vi "Contrast.vi"(4 "Burst Ct":i8[](array[numeric])=[1, 3, 5, 10, 20], 6 "CA Threshold":i16=62, 8 "File Name In":string, 9 "Voltage Steps":sgl[](array[numeric])=[100.0] format="%_3g", 10 "Motion Settings":T1={"No Motion?"=FALSE, "Motion System"=enum."NI 735x", "Motion Bd ID"=1, "Motion Profile"="SMAC1", "# Axis"=1, "Reverse Z axis?"=TRUE, "SMAC Axis"=0, "scan pair"=enum."y-(x) scan", "RT fps"=6.0, "Steps per mm"=[1000, 1000, 1000, 1000], "Motor Parameters"={"velocity ct/s"=[10000.0, 10000.0, 10000.0, 50000.0], "accel ct/s^2"=[50000.0, 50000.0, 50000.0, 200000.0]}, "One Way Scan"=FALSE, "Reverse One Way Scan"=FALSE, "Global Position (mm)"=[], "Plane"=0, "Distance between\nscan lines (um)"=0.0, "Distance between\nscan planes (um)"=0.0, "number of scan planes"=1, "Total steps in line"=0, "Xtra plane\ndistance  (um)"=100, "Xtra planes "=1, "Add Axis"=FALSE, "overshoot cts"=200, "BKPT Shift"=0, "Scan Start Time (ms)"=0, "ESP VISA"="GPIB::1::INSTR", "3rd Axis"=1, "GL Ref Out"=refnum, "Galil Address"=""} {"3rd Axis" items=["x", "y", "z", "w"]; "Xtra planes" min=1; "Xtra plane\ndistance  (um)" min=0; "Distance between\nscan planes (um)" format="%.2f"; "Distance between\nscan lines (um)" format="%.2f"; "SMAC Axis" items=["None"=0, "Axis 1"=1, "Axis 2"=2, "Axis 3"=3, "Axis 4"=4, "Axis 5"=5, "Axis 6"=6, "Axis 7"=7, "Axis 8"=8, "Vector Space 1"=17, "Vector Space 2"=18, "Vector Space 3"=19, "Vector Space 4"=20]; "Motion Bd ID" min=1 max=32 step=1}, 11 "Digitizer Settings":T5={"Digitizer delay (us) "=0.0, "rf points per line"=2048, "lines per plane"=128, "Samp Rate (Hz)"=100000000.0, "Additional dig delay (us)"=0.0, "Voltage Scale"=0.4, "Pre-Looks"=0, "Offset delay (us)"=0.0, "bits A/D"=8, "Avg Num"=1, "DigTimeOut"=5.0, "Rel Dig Delay"=0.0, "Dig Ch"=0, "LeCroyCluster"={"LeCroy Channels"=[TRUE, FALSE, FALSE, FALSE], "LC read pt offset"=0.0, "Sweep Avg"=FALSE}, "Main Digitizer"=enum."NI Digitizer", "Dig Config"=enum."Single channel", "Digitizer ID Cluster"={"Acqiris/Alazar/SP ID"=[], "NI Instr Handles"=[], "LeCroy VISA"="", "GaGe Handle"={"Handle"=0, "Sample size"=0, "Resolution"=0, "Offset"=0, "Channels"=0, "Boards"=0}, "ATS Ref"="ATS9350", "Acqiris Address"=["PCI::INSTR0"], "ADQRef"=refnum, "adq_cu_ptr"=refnum}, "Trigger Settings"={"Trig Source"=1, "Trig Coupling"=0, "Trig Slope"=0, "Level (mV)"=1500.0}, "Bulk Acq"=FALSE, "Bulk Start Indexes"=[], "Data Ref RF"=refnum, "NI ID/Channel"=[], "Total Dig CH"=1, "Xtra Ann Trig delay (us)"=10.0, "Fix Z Delay?"=FALSE, "One Way Transmission?"=FALSE, "Data Ref Log"=refnum} {"Trigger Settings"."Trig Slope" items=["Positive", "Negative"]; "Trigger Settings"."Level (mV)" format="%.2f"; "Trigger Settings"."Trig Coupling" items=["DC 1 MOhm", "AC 1 MOhm", "DC 50 Ohm", "AC 50 Ohm"]; "Trigger Settings"."Trig Source" items=["Chan 1", "External"]; "Rel Dig Delay" format="%.2f"; "DigTimeOut" format="%.2f"; "Avg Num" min=1; "Offset delay (us)" format="%.2f"; "Additional dig delay (us)" format="%.2f"; "Digitizer delay (us)" format="%.2f"}) -> (1 "Scan Params":T9={"File Name"="", "Keep?"=FALSE, "Synth Foc?"=FALSE, "Microscopy Scan Mode"=enum."Overview Scan"}, 2 "low %":dbl, 3 "clip%":dbl)   [LabVIEW 2022 SP3]
uses:
  -ScanSystem/Controls/ScanParams.ctl
  Digitizers/-DigitizerRoutines/DigitizerSettings.ctl
  Digitizers/-DigitizerRoutines/Digitizer.ctl
  Digitizers/-DigitizerRoutines/DigConfig.ctl
  Digitizers/-DigitizerRoutines/DigitizerID.ctl
  C:/Windows/System32/ADQAPI_dotNet_helper.dll
  Motion Controllers/NI_controller/-NI_MotionRoutines/MotionParameters.ctl
  Motion Controllers/NI_controller/-NI_MotionRoutines/MotionSys.ctl
  Motion Controllers/-MotionRoutines/ScanAxis.ctl
  Motion Controllers/-MotionRoutines/3rdAxis.ctl
  Motion Controllers/-MotionRoutines/MotionGlobals.vi
  <instrlib>/Acqiris Dx/Acqiris Dx.lvlib
  Digitizers/Acqiris/-AcqirisRoutines/VScaleInfoAcq.vi
  <instrlib>/niScope/Acquire/Fetch/niScope Multi Fetch Binary 8.vi
  Digitizers/NI Digitizer/-NI Digitizer VI Library/VScaleInfoNI.vi
  Pulsers/PulserGlobals.vi
  <vilib>/Utility/file.llb/Write Delimited Spreadsheet (I64).vi
  <vilib>/Utility/file.llb/Read Delimited Spreadsheet (string).vi
  <vilib>/Utility/file.llb/Write Delimited Spreadsheet (string).vi
panel:
  out "try":i32=100
  in  "M-mode Subset":i32=20
  # "1-D and 2-D B scan settings"
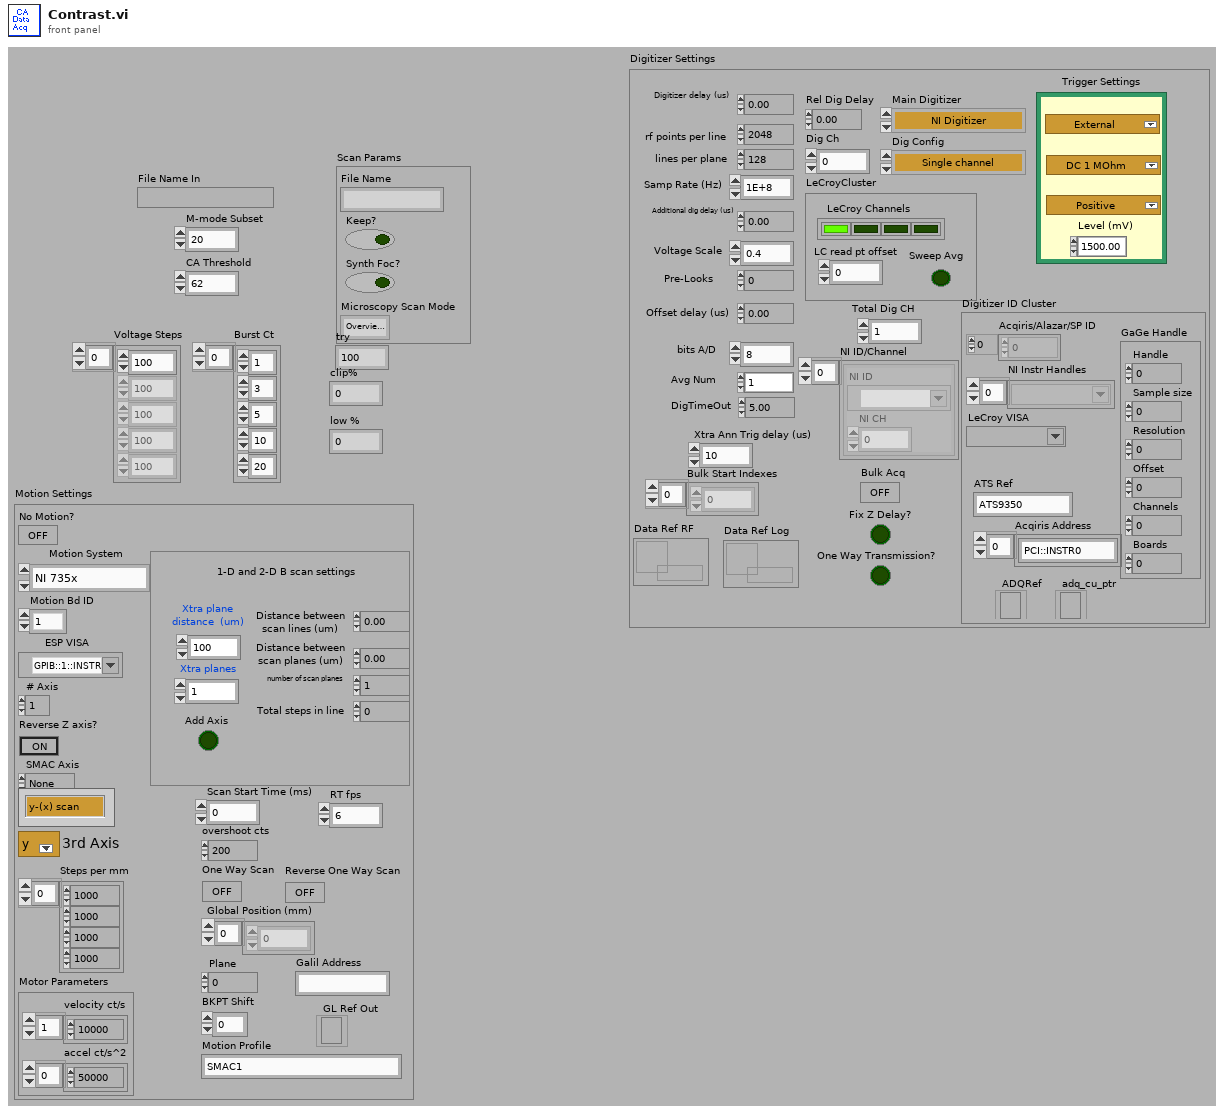
[diagram p1: front panel]
types:
  T1 = typedef "MotionParameters.ctl" = cluster{"No Motion?":bool, "Motion System":T2, "Motion Bd ID":u8, "Motion Profile":string, "# Axis":i8, "Reverse Z axis?":bool, "SMAC Axis":u16, "scan pair":T3, "RT fps":sgl, "Steps per mm":i32[], "Motor Parameters":cluster{"velocity ct/s":dbl[], "accel ct/s^2":dbl[]}, "One Way Scan":bool, "Reverse One Way Scan":bool, "Global Position (mm)":dbl[], "Plane":i32, "Distance between\nscan lines (um)":sgl, "Distance between\nscan planes (um)":sgl, "number of scan planes":i32, "Total steps in line":i32, "Xtra plane\ndistance  (um)":i32, "Xtra planes ":i32, "Add Axis":bool, "overshoot cts":i32, "BKPT Shift":i32, "Scan Start Time (ms)":u32, "ESP VISA":refnum<visa-resource-name>, "3rd Axis":T4, "GL Ref Out":refnum<k7>, "Galil Address":string}
  T2 = typedef "MotionSys.ctl" = enum16{"MM3000", "NI 735x", "Newport ESP", "No Motion Card", "Galil"}
  T3 = typedef "ScanAxis.ctl" = enum16{"y-(x) scan", "x-(y) scan", "z-(x) scan", "z-(y) scan", "y-(z) scan", "x-(z) scan", "w-(x) scan", "w-(y) scan", "w-(z) scan", "x-(w) scan", "y-(w) scan", "z-(w) scan"}
  T4 = typedef "3rdAxis.ctl" = u16
  T5 = typedef "DigitizerSettings.ctl" = cluster{"Digitizer delay (us) ":dbl, "rf points per line":i32, "lines per plane":i32, "Samp Rate (Hz)":dbl, "Additional dig delay (us)":dbl, "Voltage Scale":dbl, "Pre-Looks":i32, "Offset delay (us)":dbl, "bits A/D":i8, "Avg Num":i32, "DigTimeOut":sgl, "Rel Dig Delay":sgl, "Dig Ch":i32, "LeCroyCluster":cluster{"LeCroy Channels":bool[], "LC read pt offset":dbl, "Sweep Avg":bool}, "Main Digitizer":T6, "Dig Config":T7, "Digitizer ID Cluster":T8, "Trigger Settings":cluster{"Trig Source":u16, "Trig Coupling":u16, "Trig Slope":u16, "Level (mV)":dbl}, "Bulk Acq":bool, "Bulk Start Indexes":i32[], "Data Ref RF":refnum<data-value>, "NI ID/Channel":cluster{"NI ID":refnum<k15>, "NI CH":i32}[], "Total Dig CH":i32, "Xtra Ann Trig delay (us)":dbl, "Fix Z Delay?":bool, "One Way Transmission?":bool, "Data Ref Log":refnum<data-value>}
  T6 = typedef "Digitizer.ctl" = enum16{"Acqiris Digitizer", "NI Digitizer", "LeCroy", "GaGe", "AlazarTech", "No Digitizer", "Teledyne"}
  T7 = typedef "DigConfig.ctl" = enum16{"Single channel", "2 Chans w/ 2 Acqiris", "2 Chans w/ 1 Acqiris", "5-CH Pulser New", "5-CH pulser w/ ann array", "5-pass style ann array", "Empty"}
  T8 = typedef "DigitizerID.ctl" = cluster{"Acqiris/Alazar/SP ID":u32[], "NI Instr Handles":refnum<k15>[], "LeCroy VISA":refnum<visa-resource-name>, "GaGe Handle":cluster{"Handle":u32, "Sample size":u32, "Resolution":i32, "Offset":i32, "Channels":u32, "Boards":u32}, "ATS Ref":string, "Acqiris Address":string[], "ADQRef":refnum<k24>, "adq_cu_ptr":refnum<k24>}
  T9 = typedef "ScanParams.ctl" = cluster{"File Name":string, "Keep?":bool, "Synth Foc?":bool, "Microscopy Scan Mode":enum32{"Level X", "Level Y", "Overview Scan", "Detailed Scan", "V-Z Scan"}}
  T10 = enum32{"Level X", "Level Y", "Overview Scan", "Detailed Scan", "V-Z Scan"}
  T11 = cluster{"Therapy frequency (MHz)":dbl, "Therapy amplitude (mV)":dbl, "time therapy on (s)":dbl, "Therapy Delay (ms) ":dbl, "Time (s)":dbl}
  T12 = cluster{"Voltage Scale":i16, "Offset":dbl, "Coupling":u16}
  T13 = cluster{"actualSamples":i32, "absoluteInitialX":dbl, "relativeInitialX":dbl, "xIncrement":dbl, "offset":dbl, "gain":dbl, "reserved1":dbl, "reserved2":dbl}[]
  T14 = cluster{"actualSamples":i32, "absoluteInitialX":dbl, "relativeInitialX":dbl, "xIncrement":dbl, "offset":dbl, "gain":dbl, "reserved1":dbl, "reserved2":dbl}
  T15 = cluster{"Voltage Scale":dbl, "Offset":dbl, "Coupling":u16}
  T16 = cluster{sgl, "Gain [dB]  ":sgl, "Atten (dB)":sgl}
  T17 = cluster{"File Name In":string, bool, bool, "Microscopy Scan Mode":enum32{"Level X", "Level Y", "Overview Scan", "Detailed Scan", "V-Z Scan"}}
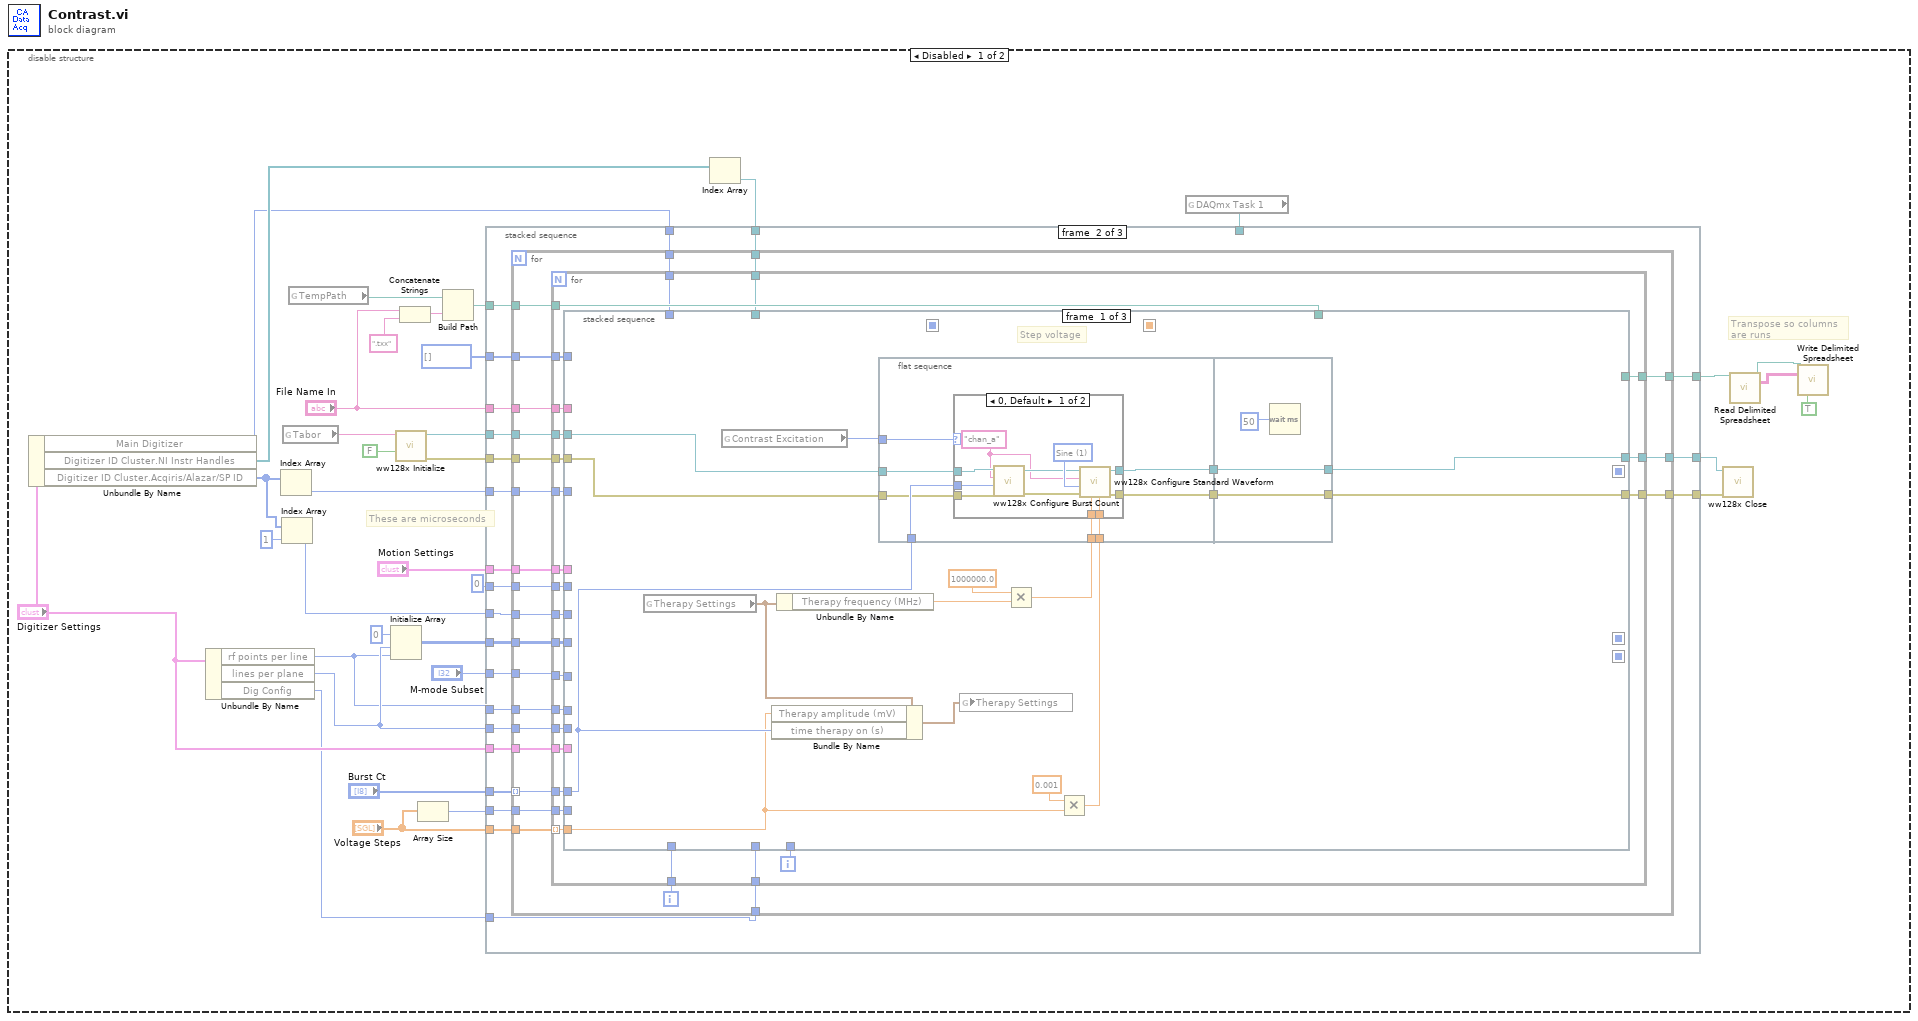
[diagram p0: block diagram]
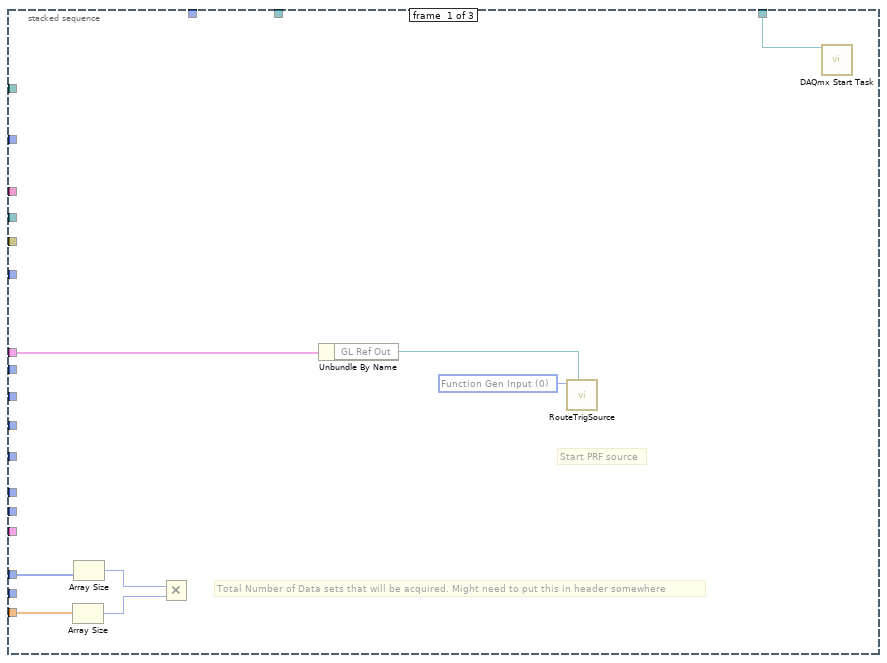
[diagram p2: hidden frame]
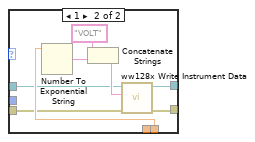
[diagram p3: hidden frame]
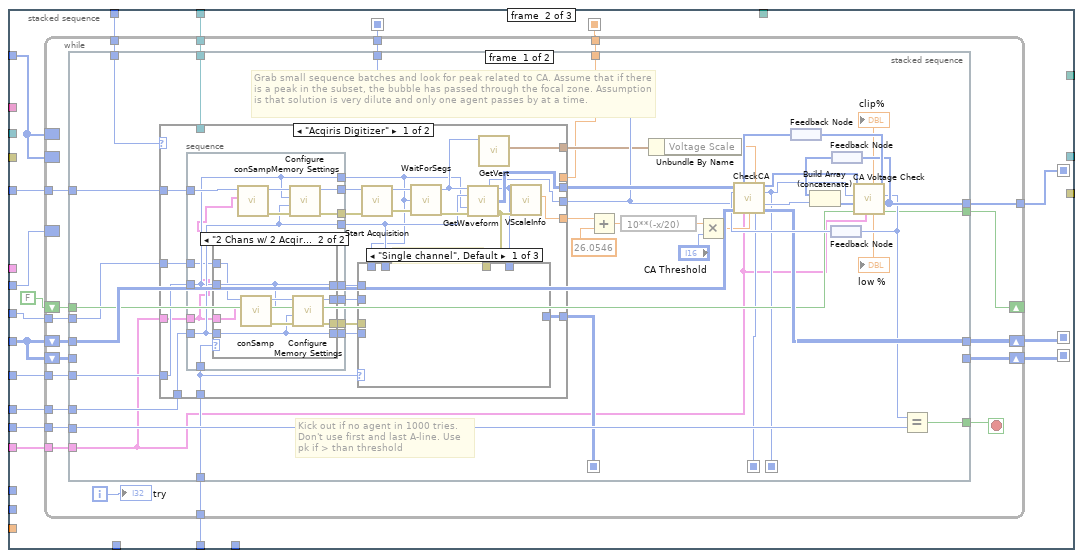
[diagram p4: hidden frame]
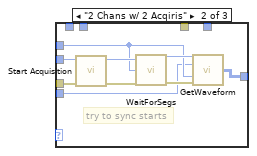
[diagram p5: hidden frame]
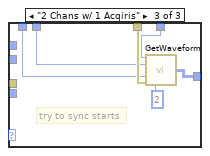
[diagram p6: hidden frame]
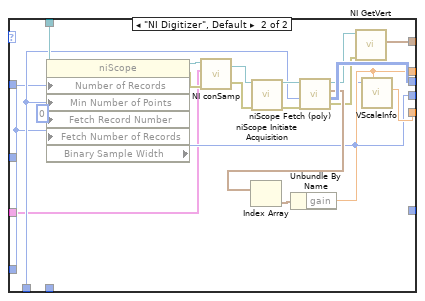
[diagram p8: hidden frame]
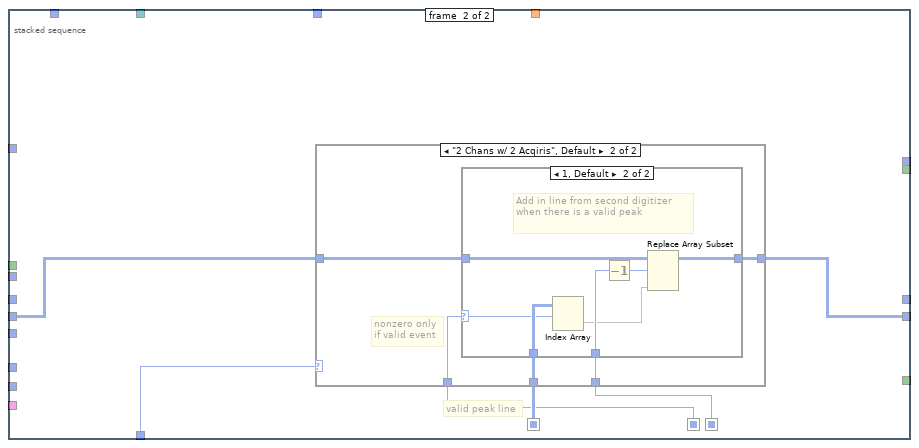
[diagram p9: hidden frame]
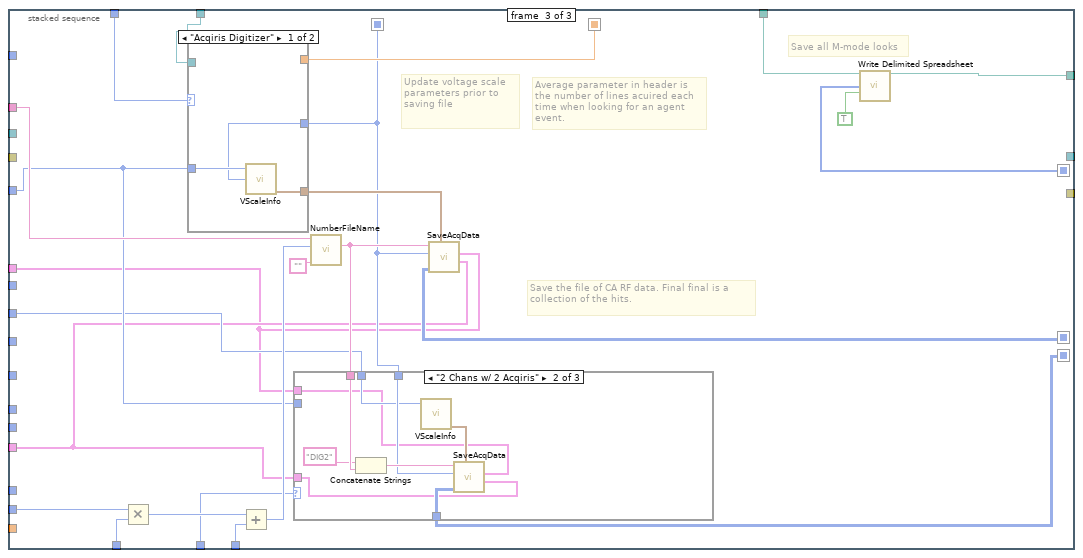
[diagram p12: hidden frame]
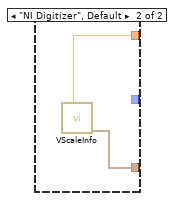
[diagram p13: hidden frame]
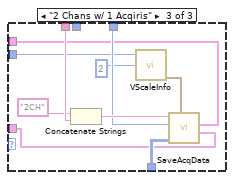
[diagram p15: hidden frame]
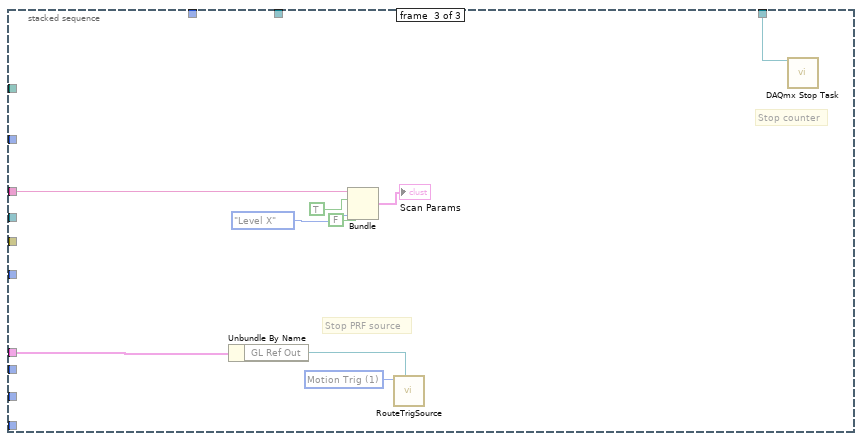
[diagram p16: hidden frame]
diagram:
  n1 = disable-structure shown="Disabled" {
    frame Disabled {
      # "Transpose so columns are runs"
      # "These are microseconds"
      n2 = Unbundle By Name("Digitizer Settings") -> ("Main Digitizer"=w5:T6, "Digitizer ID Cluster.NI Instr Handles"=w12:refnum<k15>[], "Digitizer ID Cluster.Acqiris/Alazar/SP ID"=w10:u32[])
      n3 = Unbundle By Name("Digitizer Settings") -> ("rf points per line"=w7:i32, "lines per plane"=w8:i32, "Dig Config"=w4:T7)
      n4 = Index Array(array=w10) -> (element=w13:u32)  [unwired: 1 in]
      n5 = Index Array(array=w10, index=1) -> (element=w9:u32)
      n6 = global read "PulserGlobals.vi" "Tabor"() -> (w3:string)
      n7 = global read "MotionGlobals.vi" "TempPath"() -> (w14:path)
      n8 = Initialize Array(i16 0, w8, w7) -> (w35:i16[][])
      n9 = call <instrlib>:"ww128x Initialize.vi"("reset device (Yes)"=FALSE ("reset device"), "resource name"=w3) -> ("error out"=w17:errorcluster, "instrument handle out"=w16:refnum<k15>)  [unwired: 2 in, 6 out]
      n10 = Concatenate Strings("File Name In", ".txx") -> (w23:string)
      n11 = Array Size(array="Voltage Steps") -> (size(s)=w29:i32)
      n12 = Build Path(base path=w14, name or relative path=w23) -> (appended path=w21:path)
      n13 = Index Array(array=w12) -> (element=w15:refnum<k15>)  [unwired: 1 in]
      n14 = global read "MotionGlobals.vi" "DAQmx Task 1"() -> (w32:refnum<k21>)
      n15 = stacked-sequence {
        tunnel: w13 -> [_ w67 _]
        tunnel: w7 -> [_ w66 _]
        tunnel: "M-mode Subset" -> [_ w65 _]
        tunnel: w35 -> [_ w64 _]
        tunnel: 0 -> [_ w63 _]
        tunnel: w8 -> [_ w62 _]
        tunnel: "File Name In" -> [_ w61 w395]
        tunnel: w32 -> [w44 _ w398]
        tunnel: i32[] [] -> [_ w60 _]
        tunnel: "Burst Ct" -> [w42 w59 _]
        tunnel: "Voltage Steps" -> [w43 w58 _]
        tunnel: w29 -> [_ w57 _]
        tunnel: [_ w56 _] -> w28
        tunnel: w21 -> [_ w55 _]
        tunnel: [_ w54 _] -> w20
        tunnel: [_ w53 _] -> w19
        tunnel: w17 -> [_ w52 _]
        tunnel: w16 -> [_ w51 _]
        tunnel: w5 -> [_ w50 _]
        tunnel: w15 -> [_ w49 _]
        tunnel: w9 -> [_ w48 _]
        tunnel: "Digitizer Settings" -> [_ w47 _]
        tunnel: w4 -> [_ w46 _]
        tunnel: "Motion Settings" -> [w38 w45 w391]
        frame #0 {
          w39 = u16 0 items=["Function Gen Input", "Motion Trig", "Internal RT Motion Trig", "Internal CTR 1 Output"] ("Trig Source")
          # "Total Number of Data sets that will be acquired. Might need to put this in header somewhere"
          # "Start PRF source"
          n16 = Array Size(array=w43) -> (size(s)=w40:i32)
          n17 = Array Size(array=w42) -> (size(s)=w41:i32)
          n18 = Multiply(x=w41, y=w40) -> ()  [unwired: 1 out]
          n19 = Unbundle By Name(w38) -> ("GL Ref Out"=w37:refnum<k7>)
          n20 = call "RouteTrigSource.vi"("Galil.IGalil"=w37, "Trig Source"=w39) -> ()  [unwired: 9 in, 1 out]
          n21 = call <vilib>:"DAQmx Start Task.vi"("task/channels in"=w44) -> ()  [unwired: 1 in, 14 out]
        }
        frame #1 {
          n22 = for {
            tunnel: w67 -> [w91]
            tunnel: w66 -> [w90]
            tunnel: w65 -> [w89]
            tunnel: w64 -> [w88]
            tunnel: w63 -> [w87]
            tunnel: w62 -> [w86]
            tunnel: w61 -> [w85]
            tunnel: w60 -> [w84]
            tunnel: w59 -> [w83] mode=indexing
            tunnel: w58 -> [w82]
            tunnel: w57 -> [w81]
            tunnel: [w79] -> w56
            tunnel: w55 -> [w78]
            tunnel: [w77] -> w54
            tunnel: [w76] -> w53
            tunnel: w52 -> [w75]
            tunnel: w51 -> [w74]
            tunnel: w50 -> [w73]
            tunnel: w49 -> [w72]
            tunnel: w46 -> [w71]
            tunnel: w48 -> [w70]
            tunnel: w47 -> [w69]
            tunnel: w45 -> [w68]
            i -> [w80]
            n23 = for {
              tunnel: w91 -> [w116]
              tunnel: w89 -> [w115]
              tunnel: w90 -> [w114]
              tunnel: w88 -> [w113]
              tunnel: w87 -> [w112]
              tunnel: w86 -> [w111]
              tunnel: w85 -> [w110]
              tunnel: w84 -> [w109]
              tunnel: w83 -> [w108]
              tunnel: w82 -> [w107] mode=indexing
              tunnel: w81 -> [w106]
              tunnel: w80 -> [w105]
              tunnel: [w103] -> w79
              tunnel: w78 -> [w102]
              tunnel: [w101] -> w77
              tunnel: [w100] -> w76
              tunnel: w75 -> [w99]
              tunnel: w74 -> [w98]
              tunnel: w73 -> [w97]
              tunnel: w72 -> [w96]
              tunnel: w71 -> [w95]
              tunnel: w70 -> [w94]
              tunnel: w69 -> [w93]
              tunnel: w68 -> [w92]
              i -> [w104]
              n24 = stacked-sequence {
                seq-local: [_ w176 _] -> [_ _ w363]
                seq-local: [_ w174 _] -> [_ _ w345]
                seq-local: [_ w168 _] -> [_ _ w356]
                seq-local: [_ w166 _] -> [_ _ w351]
                seq-local: [_ w165 _] -> [_ _ w346]
                tunnel: w116 -> [_ w179 w347]
                tunnel: w115 -> [_ w178 _]
                tunnel: w114 -> [_ w180 _]
                tunnel: w113 -> [_ w169 _]
                tunnel: w112 -> [_ w177 _]
                tunnel: w111 -> [_ w167 _]
                tunnel: w110 -> [_ _ w364]
                tunnel: w109 -> [_ w175 _]
                tunnel: w108 -> [w119 _ _]
                tunnel: w107 -> [w118 _ _]
                tunnel: w106 -> [_ _ w362]
                tunnel: w105 -> [_ _ w361]
                tunnel: w104 -> [_ _ w360]
                tunnel: w102 -> [_ _ w357]
                tunnel: [_ _ w354] -> w103
                tunnel: [w127 _ _] -> w101
                tunnel: [w125 _ _] -> w100
                tunnel: w99 -> [w124 _ _]
                tunnel: w98 -> [w123 _ _]
                tunnel: w97 -> [_ w172 w349]
                tunnel: w96 -> [_ w171 w350]
                tunnel: w95 -> [_ w170 w353]
                tunnel: w94 -> [_ w164 w344]
                tunnel: w93 -> [_ w163 w343]
                tunnel: w92 -> [_ _ w342]
                frame #0 {
                  # "Step voltage"
                  n25 = global read "PulserGlobals.vi" "Therapy Settings"() -> (w120:T11)
                  n26 = global read "PulserGlobals.vi" "Contrast Excitation"() -> (w122:u16)
                  n27 = Bundle By Name(cluster=w120, "Therapy amplitude (mV)"=w118, "time therapy on (s)"=w119) -> (w117:T11)
                  n28 = Unbundle By Name(w120) -> ("Therapy frequency (MHz)"=w121:dbl)
                  n29 = flat-sequence {
                    tunnel: w119 -> [w137]
                    tunnel: w130 -> [w140]
                    tunnel: w129 -> [w139]
                    tunnel: w122 -> [w138]
                    tunnel: [w136] -> w128
                    tunnel: [w135] -> w126
                    tunnel: w124 -> [w134]
                    tunnel: w123 -> [w133]
                    tunnel: w128 -> [w161]
                    tunnel: [w161] -> w127
                    tunnel: [w160] -> w125
                    tunnel: w126 -> [w160]
                    frame #0 {
                      n30 = case shown="0, Default" w138 {
                        tunnel: [w151 w159] -> w135
                        tunnel: w140 -> [w150 w155]
                        tunnel: w139 -> [w149 _]
                        tunnel: w137 -> [w145 _]
                        tunnel: [w144 w154] -> w136
                        tunnel: w134 -> [w142 w153]
                        tunnel: w133 -> [w143 w152]
                        frame 0, Default {
                          w141 = "chan_a" ("channel name (\"CHAN_A\")")
                          w148 = 1 items=["Sine"=1, "Square"=2, "Triangle"=3, "Ramp Up"=4, "Ramp Down"=5, "DC"=6, "Ramp"=1001, "Pulse"=1005, "Sync"=1002, "Gaussian"=1003, "Exponential"=1004, "Noise"=1006] ("waveform")
                          n31 = call <instrlib>:"ww128x Configure Burst Count.vi"("error in (no error)"=w142, "burst count (2)"=w145, "channel name (\"CHAN_A\")"=w141, "instrument handle"=w143) -> ("error out"=w147:errorcluster, "instrument handle out"=w146:refnum<k15>)  [unwired: 6 out]
                          n32 = call <instrlib>:"ww128x Configure Standard Waveform.vi"("amplitude"=w150, "frequency"=w149, "error in (no error)"=w147, "waveform"=w148, "channel name"=w141, "instrument handle"=w146) -> ("error out"=w144:errorcluster, "instrument handle out"=w151:refnum<k15>)  [unwired: 2 in, 2 out]
                        }
                        frame 1 {
                          n33 = Number To Exponential String(number=w155) -> (E-format string=w157:string)  [unwired: 3 out]
                          n34 = Concatenate Strings("VOLT" ("string"), w157) -> (w156:string)
                          n35 = call <instrlib>:"ww128x Write Instrument Data.vi"("error in (no error)"=w153, "write buffer"=w156, "instrument handle"=w152) -> ("error out"=w154:errorcluster, "instrument handle out"=w159:refnum<k15>)  [unwired: 7 out]
                        }
                      }
                    }
                    frame #1 {
                      n36 = Wait (ms)(milliseconds to wait=50) -> ()  [unwired: 1 out]
                    }
                  }
                  n37 = global write "PulserGlobals.vi" "Therapy Settings"(w117) -> ()
                  n38 = Multiply(x=1000000.0, y=w121) -> (x*y=w129:dbl)
                  n39 = Multiply(x=0.001, y=w118) -> (x*y=w130:dbl)
                }
                frame #1 {
                  n40 = while {
                    tunnel: w180 -> [w197]
                    tunnel: w179 -> [w200]
                    tunnel: w178 -> [w196]
                    shift-right: [w194] -> w176
                    shift-left: w169 -> [w199]
                    tunnel: w167 -> [w186]
                    border: w177 -> [_]
                    border: w175 -> [_]
                    border: w175 -> [_]
                    tunnel: [w190] -> w174
                    shift-right: [w192] -> _
                    shift-left: FALSE -> [w193]
                    tunnel: w172 -> [w191]
                    tunnel: w171 -> [w189]
                    tunnel: w170 -> [w188]
                    shift-right: [w184] -> w166
                    shift-left: w169 -> [w185]
                    tunnel: [w195] -> w168
                    tunnel: [w183] -> w165
                    tunnel: w164 -> [w182]
                    tunnel: w163 -> [w181]
                    i -> [w187]
                    stop <- w198 stop-if-true
                    n41 = stacked-sequence {
                      seq-local: [w206 _] -> [_ w325]
                      seq-local: [w205 _] -> [_ w327]
                      seq-local: [w204 _] -> [_ w323]
                      tunnel: w200 -> [w239 _]
                      tunnel: w199 -> [w238 _]
                      tunnel: [w237 _] -> w198
                      tunnel: w186 -> [w236 _]
                      tunnel: w197 -> [w235 _]
                      tunnel: w196 -> [w234 _]
                      tunnel: [w227 _] -> w195
                      tunnel: [w225 _] -> w194
                      tunnel: w193 -> [w216 _]
                      tunnel: [w215 _] -> w192
                      tunnel: w191 -> [w213 _]
                      tunnel: [w212 _] -> w190
                      tunnel: w189 -> [w210 _]
                      tunnel: w188 -> [w207 w324]
                      tunnel: w185 -> [_ w326]
                      tunnel: [_ w322] -> w184
                      tunnel: [w203 _] -> w183
                      tunnel: w182 -> [w202 _]
                      tunnel: w181 -> [w201 _]
                      frame #0 {
                        # "Grab small sequence batches and look for peak related to CA. Assume that if there is a peak in the subset, the bubble has passed through the focal zone. Assumption is that solution is very dilute and only one agent passes by at a time."
                        # "Kick out if no agent in 1000 tries. Don't use first and last A-line. Use pk if > than threshold"
                        n42 = case shown="\"Acqiris Digitizer\"" w213 {
                          tunnel: w239 -> [w262 _]
                          tunnel: w235 -> [w254 w309]
                          tunnel: w234 -> [w249 w308]
                          tunnel: [w256 w317] -> w233
                          tunnel: [w242 w303] -> w212
                          tunnel: [w259 w321] -> w211
                          tunnel: [w255 w318] -> w219
                          tunnel: w210 -> [_ w310]
                          tunnel: w207 -> [w248 _]
                          tunnel: [w253 _] -> w206
                          tunnel: [_ w304] -> w203
                          tunnel: w202 -> [w241 _]
                          tunnel: w201 -> [w240 w302]
                          frame "Acqiris Digitizer" {
                            # "2nd digitizer acq"
                            n43 = stacked-sequence {
                              tunnel: w262 -> [w291]
                              tunnel: [w290] -> w261
                              tunnel: [w289] -> w260
                              tunnel: w254 -> [w286]
                              tunnel: [w288] -> w252
                              tunnel: [w287] -> w251
                              tunnel: [w286] -> w244
                              tunnel: [w285] -> w243
                              tunnel: [w283] -> w250
                              tunnel: w249 -> [w285]
                              tunnel: w248 -> [w284]
                              tunnel: [w282] -> w247
                              tunnel: w241 -> [w281]
                              tunnel: w240 -> [w280]
                              frame #0 {
                                n44 = case shown="\"2 Chans w/ 2 Acqiris\"" w284 {
                                tunnel: [_ w301] -> w288
                                tunnel: [_ w298] -> w287
                                tunnel: w286 -> [_ w296]
                                tunnel: w285 -> [_ w297]
                                tunnel: [_ w297] -> w283
                                tunnel: [_ w296] -> w282
                                tunnel: w281 -> [_ w295]
                                tunnel: w280 -> [_ w294]
                                frame "Single channel", Default {
                                }
                                frame "2 Chans w/ 2 Acqiris" {
                                n45 = call "conSamp.vi"("Digitizer Settings"=w294, "InstrumentID"=w295) -> ("error out"=w299:errorcluster, "DUP ID"=w300:u32)  [unwired: 2 in]
                                n46 = call <instrlib>:"Configure Memory Settings.vi"("error in (no error)"=w299, "Number of Samples (1000)"=w296, "Number of Segments (1)"=w297, "Instrument ID"=w300) -> ("error out"=w298:errorcluster, "dup Instrument ID"=w301:u32)  [unwired: 2 out]
                                }
                                }
                                n47 = call "conSamp.vi"("Digitizer Settings"=w280, "InstrumentID"=w291) -> ("error out"=w292:errorcluster, "DUP ID"=w293:u32)  [unwired: 2 in]
                                n48 = call <instrlib>:"Configure Memory Settings.vi"("error in (no error)"=w292, "Number of Samples (1000)"=w286, "Number of Segments (1)"=w285, "Instrument ID"=w293) -> ("error out"=w289:errorcluster, "dup Instrument ID"=w290:u32)  [unwired: 2 out]
                              }
                            }
                            n49 = call <instrlib>:"Start Acquisition.vi"("error in (no error)"=w260, "Instrument ID"=w261) -> ("error out"=w263:errorcluster, "dup Instrument ID"=w264:u32)  [unwired: 2 in]
                            n50 = call "WaitForSegs.vi"("Acqiris ID"=w264, "lines per plane"=w243, "error in"=w263) -> ("dup Instrument ID"=w258:u32, "error out"=w257:errorcluster)  [unwired: 1 in, 2 out]
                            n51 = call "GetWaveform.vi"("Acq ID Out"=w258, "Num Samps"=w244, "Num Segs"=w243, "error in"=w257) -> ("Dig Word Size"=w242:u16, "Acq ID Out"=w245:u32, "Acquired Waveform16 bit"=w256:i16[][], "error out"=w246:errorcluster)  [unwired: 2 in, 6 out]
                            n52 = case shown="\"Single channel\", Default" w248 {
                              tunnel: [_ w273 w279] -> w253
                              tunnel: w252 -> [_ w271 _]
                              tunnel: w251 -> [_ w269 _]
                              tunnel: w250 -> [_ w266 _]
                              tunnel: w247 -> [_ w265 _]
                              tunnel: w246 -> [_ _ w278]
                              tunnel: w245 -> [_ _ w277]
                              tunnel: w244 -> [_ _ w275]
                              tunnel: w243 -> [_ _ w274]
                              frame "Single channel", Default {
                              }
                              frame "2 Chans w/ 2 Acqiris" {
                                # "try to sync starts"
                                n53 = call <instrlib>:"Start Acquisition.vi"("error in (no error)"=w269, "Instrument ID"=w271) -> ("error out"=w268:errorcluster, "dup Instrument ID"=w270:u32)  [unwired: 2 in]
                                n54 = call "WaitForSegs.vi"("Acqiris ID"=w270, "lines per plane"=w266, "error in"=w268) -> ("dup Instrument ID"=w272:u32, "error out"=w267:errorcluster)  [unwired: 1 in, 2 out]
                                n55 = call "GetWaveform.vi"("Acq ID Out"=w272, "Num Samps"=w265, "Num Segs"=w266, "error in"=w267) -> ("Acquired Waveform16 bit"=w273:i16[][])  [unwired: 2 in, 9 out]
                              }
                              frame "2 Chans w/ 1 Acqiris" {
                                # "try to sync starts"
                                n56 = call "GetWaveform.vi"("Acq ID Out"=w277, "Num Samps"=w275, "Num Segs"=w274, "error in"=w278, "Channel"=2) -> ("Acquired Waveform16 bit"=w279:i16[][])  [unwired: 1 in, 9 out]
                              }
                            }
                            n57 = call "GetVert.vi"("InstrumentID"=w258) -> ("V scale"=w259:T12)  [unwired: 3 in, 3 out]
                            n58 = call-poly "VScaleInfo.vi"("Instrument ID"=w245, "error in (no error)"=w246) -> ("vGain (dB)"=w255:dbl)  [unwired: 1 in, 7 out]
                          }
                          frame "NI Digitizer", Default {
                            n59 = property class="niScope"(reference=w310, "Number of Records"=w308, "Min Number of Points"=w309, "Fetch Record Number"=0, "Fetch Number of Records"=w308) -> (reference out=w314:refnum<k15>, error out=w311:errorcluster, "Binary Sample Width"=w303:i32)  [unwired: 1 in]
                            n60 = call "NI conSamp.vi"("error in"=w311, "Digitizer Settings"=w302, "InstrumentID"=w314) -> ("error out"=w312:errorcluster, "DUP ID"=w313:refnum<k15>)  [unwired: 1 in]
                            n61 = call <instrlib>:"niScope Initiate Acquisition.vi"("instrument handle"=w313, "error in"=w312) -> ("instrument handle out"=w320:refnum<k15>, "error out"=w319:errorcluster)  [unwired: 1 in, 11 out]
                            n62 = call-poly <instrlib>:"niScope Fetch (poly).vi"("error in"=w319, "numSamples"=w309, "instrument handle"=w320) -> ("error out"=w305:errorcluster, "wfm"=w317:i8[][], "wfm info"=w307:T13, "instrument handle out"=w315:refnum<k15>)  [unwired: 2 in, 3 out]
                            n63 = Index Array(array=w307) -> (element=w306:T14)  [unwired: 1 in]
                            n64 = Unbundle By Name(w306) -> ("gain"=w304:dbl)
                            n65 = call "NI GetVert.vi"("error in"=w305, "InstrumentID"=w315) -> ("V scale"=w321:T15)  [unwired: 1 in, 4 out]
                            n66 = call-poly "VScaleInfo.vi"("A/D bits"=w303, "gain"=w304) -> ("vGain (dB)"=w318:dbl)  [unwired: 1 in, 7 out]
                          }
                        }
                        n67 = Add(x=w219, y=26.0546) -> (x+y=w218:dbl)
                        n68 = expression code="10**(-x/20)"(w218) -> (w209:dbl)
                        n69 = Unbundle By Name(w211) -> ("Voltage Scale"=w220:dbl)
                        n70 = Multiply(x=w209, y="CA Threshold") -> (x*y=w217:dbl)
                        n71 = feedback #1() -> (w222:i32[])
                        n72 = feedback #2() -> (w232:i32)
                        n73 = call "CheckCA.vi"("data"=w233, "valid peak in"=w222, "Voltage Scale"=w220, "count in"=w232, "Dig Word Size"=w212, "fill array"=w238, "Digitizer Settings"=w201, "CA Threshold"=w217) -> ("valid peak out"=w221:i32[], "count out"=w205:i32, "All peaks"=w231:i32, "valild peak line"=w204:i32, "fill out"=w225:i16[][])  [unwired: 3 in]
                        n74 = feedback #3() -> (w230:i32[])
                        n75 = Build Array (concatenate)(w230, w231) -> (w228:i32[])
                        n76 = call "CA Voltage Check.vi"("Digitizer Settings"=w201, "Up Once?"=w216, "All Peak in"=w228, "count in"=w205, "valid peak in"=w221) -> ("Up Once Out"=w215:bool, "All Peak Out"=w227:i32[], "count out"=w226:i32, "valid peak out"=w229:i32[], "low %"=→"low %":dbl, "clip%"=→"clip%":dbl)  [unwired: 1 in]
                        n77 = feedback-in #1(w229) -> ()
                        n78 = feedback-in #2(w226) -> ()
                        n79 = feedback-in #3(w227) -> ()
                        n80 = Equal?(x=w226, y=w236) -> (x = y?=w237:bool)
                      }
                      frame #1 {
                        # "valid peak line"
                        n81 = case shown="\"2 Chans w/ 2 Acqiris\", Default" w324 {
                          tunnel: w327 -> [_ w333]
                          tunnel: w326 -> [w328 w332]
                          tunnel: w325 -> [_ w331]
                          tunnel: w323 -> [_ w330]
                          tunnel: [w328 w329] -> w322
                          frame "Single channel" {
                          }
                          frame "2 Chans w/ 2 Acqiris", Default {
                            # "nonzero only if valid event"
                            n82 = case shown="1, Default" w330 {
                              selector: w330 -> [_ w336]
                              tunnel: w333 -> [_ w341]
                              tunnel: w332 -> [w334 w340]
                              tunnel: w331 -> [_ w338]
                              tunnel: [w334 w335] -> w329
                              frame 0 {
                              }
                              frame 1, Default {
                                # "Add in line from second digitizer when there is a valid peak"
                                n83 = Index Array(array=w338, index (row)=w336) -> (element=w337:i16[])  [unwired: 1 in]
                                n84 = Decrement(x=w341) -> (x-1=w339:i32)
                                n85 = Replace Array Subset(array=w340, new element=w337, index (row)=w339) -> (w335:i16[][])  [unwired: 1 in]
                              }
                            }
                          }
                        }
                      }
                    }
                    "try" <- w187
                  }
                }
                frame #2 {
                  # "Update voltage scale parameters prior to saving file"
                  # "Average parameter in header is the number of lines acuired each time when looking for an agent event."
                  # "Save all M-mode looks"
                  # "Save the file of CA RF data. Final final is a collection of the hits."
                  n86 = Multiply(x=w362, y=w361) -> (x*y=w359:i32)
                  n87 = case shown="\"Acqiris Digitizer\"" w349 {
                    tunnel: w350 -> [_ _]
                    tunnel: [w368 w370] -> w348
                    tunnel: w347 -> [w367 _]
                    tunnel: w346 -> [_ w369]
                    tunnel: w345 -> [w366 _]
                    frame "Acqiris Digitizer" {
                      n88 = call-poly "VScaleInfo.vi"("Instrument ID"=w367, "Channel (1)"=w366) -> ("Voltage Scale"=w368:T16)  [unwired: 1 in, 7 out]
                    }
                    frame "NI Digitizer", Default {
                      n89 = call-poly "VScaleInfo.vi"("gain"=w369) -> ("Voltage Scale"=w370:T16)  [unwired: 1 in, 8 out]
                    }
                  }
                  n90 = Add(x=w359, y=w360) -> (x+y=w358:i32)
                  n91 = call "NumberFileName.vi"("String"="", "File number"=w358, "file name"=w364) -> ("Numbered File"=w352:string)  [unwired: 1 in]
                  n92 = case shown="\"2 Chans w/ 2 Acqiris\"" w353 {
                    tunnel: w352 -> [_ w379 w389]
                    tunnel: w351 -> [_ w376 w386]
                    tunnel: w345 -> [_ w375 w385]
                    tunnel: w347 -> [_ _ w382]
                    tunnel: w344 -> [_ w373 _]
                    tunnel: w343 -> [_ w372 w381]
                    tunnel: w342 -> [_ w371 w380]
                    frame "Single channel", Default {
                    }
                    frame "2 Chans w/ 2 Acqiris" {
                      n93 = Concatenate Strings("DIG2", w379) -> (w377:string)
                      n94 = call-poly "VScaleInfo.vi"("Instrument ID"=w373) -> ("Voltage Scale"=w374:T16)  [unwired: 2 in, 7 out]
                      n95 = call "SaveAcqData.vi"("Digitizer Settings"=w372, "Motion Settings"=w371, "Votage scaling"=w374, "Array"=w376, "Dig Word Size"=w375, "File Name"=w377) -> ()  [unwired: 5 in]
                    }
                    frame "2 Chans w/ 1 Acqiris" {
                      n96 = Concatenate Strings("2CH", w389) -> (w387:string)
                      n97 = call-poly "VScaleInfo.vi"("Instrument ID"=w382, "Channel (1)"=2) -> ("Voltage Scale"=w384:T16)  [unwired: 1 in, 7 out]
                      n98 = call "SaveAcqData.vi"("Digitizer Settings"=w381, "Motion Settings"=w380, "Votage scaling"=w384, "Array"=w386, "Dig Word Size"=w385, "File Name"=w387) -> ()  [unwired: 5 in]
                    }
                  }
                  n99 = call "SaveAcqData.vi"("Digitizer Settings"=w343, "Motion Settings"=w342, "Votage scaling"=w348, "Array"=w363, "Dig Word Size"=w345, "File Name"=w352) -> ()  [unwired: 5 in]
                  n100 = call-poly <vilib>:"Write Delimited Spreadsheet.vi"("file path (dialog if empty)"=w357, "1D data"=w356, "append to file? (new file:F)"=TRUE ("transpose? (no:F)")) -> ("new file path (Not A Path if cancelled)"=w354:path)  [unwired: 11 in, 1 out]
                }
              }
            }
          }
        }
        frame #2 {
          w393 = u16 1 items=["Function Gen Input", "Motion Trig", "Internal RT Motion Trig", "Internal CTR 1 Output"] ("Trig Source")
          # "Stop counter"
          # "Stop PRF source"
          n101 = Unbundle By Name(w391) -> ("GL Ref Out"=w390:refnum<k7>)
          n102 = Bundle("File Name In"=w395, TRUE, FALSE, "Microscopy Scan Mode"=T10."Level X") -> (→"Scan Params":T17)  [unwired: 1 out]
          n103 = call "RouteTrigSource.vi"("Galil.IGalil"=w390, "Trig Source"=w393) -> ()  [unwired: 9 in, 1 out]
          n104 = call <vilib>:"DAQmx Stop Task.vi"("task/channels in"=w398) -> ()  [unwired: 1 in, 14 out]
        }
      }
      n105 = call <instrlib>:"ww128x Close.vi"("error in (no error)"=w20, "instrument handle"=w19) -> ()  [unwired: 10 out]
      n106 = call-poly <vilib>:"Read Delimited Spreadsheet.vi"("file path (dialog if empty)"=w28) -> ("new file path (Not A Path if cancelled)"=w26:path, "all rows"=w2:string[][])  [unwired: 9 in, 4 out]
      n107 = call-poly <vilib>:"Write Delimited Spreadsheet.vi"("file path (dialog if empty)"=w26, "2D data"=w2, "transpose? (no:F)"=TRUE) -> ()  [unwired: 11 in, 2 out]
    }
    frame Enabled {
    }
  }
